vi "Read rioResourceName.vi"(8 "error in (no error)":errorcluster, 11 "RIOConfig in":refnum<class "RIOConfig.lvclass">) -> (0 "error out":errorcluster, 2 "rioResourceName":string="RIO0", 3 "RIOConfig out":refnum<class "RIOConfig.lvclass">)   [LabVIEW 2013, in "ComponentData.lvlib" / "RIOConfig.lvclass"]
uses:
  <userlib>/Common/Component/Application/RT/ComponentData/ConfigurationHandler/RIOConfig/RIOConfig.lvclass
  <userlib>/Common/Component/Application/RT/ComponentData/ConfigurationHandler/RIOConfig/RIOConfig.lvclass/RIOConfig.ctl
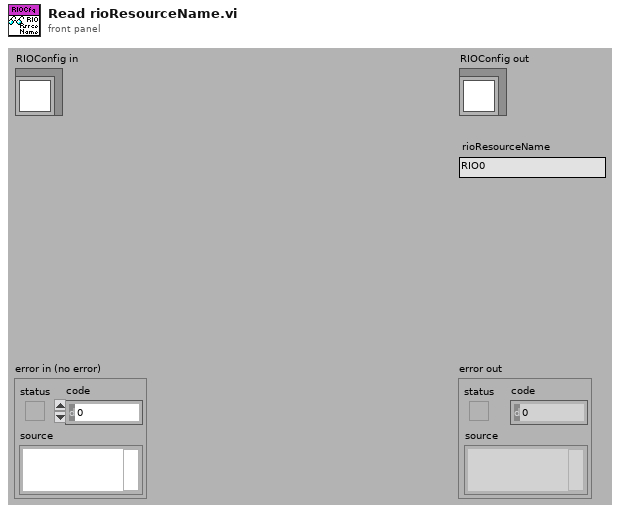
[diagram p1: front panel]
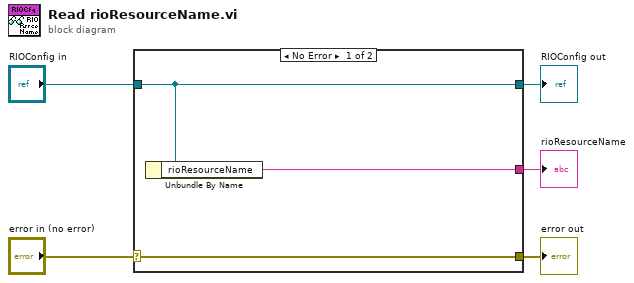
[diagram p0: block diagram]
diagram:
  n1 = case shown="No Error" "error in (no error)" {
    selector: "error in (no error)" -> [w8 w9]
    tunnel: [w8 w9] -> w4
    tunnel: [w7 w10] -> w2
    tunnel: "RIOConfig in" -> [w7 w10]
    tunnel: [w6 _] -> w1
    frame No Error {
      n2 = Unbundle By Name(w7) -> ("rioResourceName"=w6:string)
    }
    frame Error {
    }
  }
  "error out" <- w4
  "RIOConfig out" <- w2
  "rioResourceName" <- w1
